vi "FileWriterTest.vi"() -> ()   [LabVIEW 2020]
uses:
  typedefs/typedef_stage_position.ctl
  <vilib>/numeric/Random Number (Range) U64.vi
  <vilib>/numeric/sub_Random U32.vi
panel:
  in  "stop":bool
  in  "file path (use dialog)":path
  in  "Stage position":T1
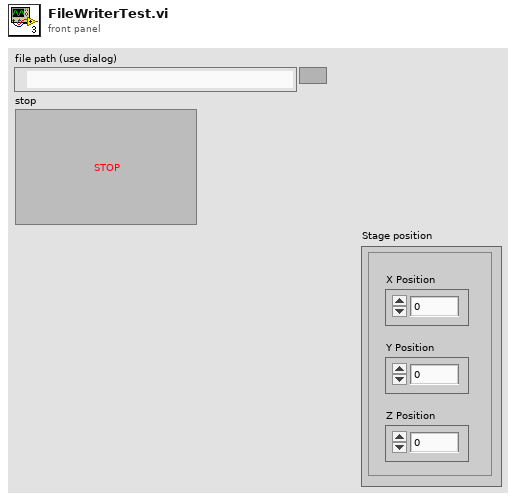
[diagram p1: front panel]
types:
  T1 = typedef "typedef_stage_position.ctl" = cluster{"X Position":dbl, "Y Position":dbl, "Z Position":dbl}
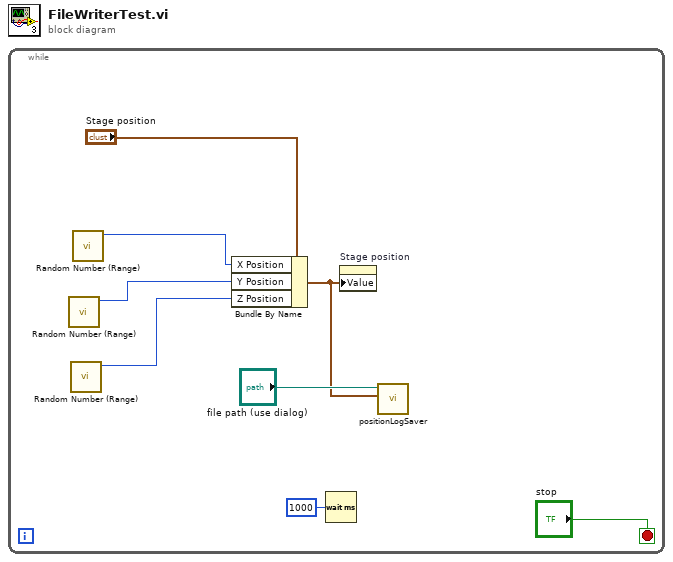
[diagram p0: block diagram]
diagram:
  n1 = while {
    stop <- "stop" stop-if-true
    n2 = call-poly <vilib>:"Random Number (Range).vi"() -> ("number"=w6:u64)  [unwired: 11 in]
    n3 = call-poly <vilib>:"Random Number (Range).vi"() -> ("number"=w5:u64)  [unwired: 11 in]
    n4 = call-poly <vilib>:"Random Number (Range).vi"() -> ("number"=w7:u64)  [unwired: 11 in]
    n5 = Bundle By Name(cluster="Stage position", "X Position"=w7, "Y Position"=w6, "Z Position"=w5) -> (w3:T1)
    n6 = Wait (ms)(milliseconds to wait=u32 1000) -> ()  [unwired: 1 out]
    n7 = property on="Stage position" class="Clust (strict)"("Value"=w3) -> ()  [unwired: 2 in, 2 out]
    n8 = call "positionLogSaver.vi"("Stage position"=w3, "file path (use dialog)"="file path (use dialog)") -> ()  [unwired: 10 in]
  }
